vi "Plural Marker.vi"(11 "Size":i32) -> (3 "Plural Mark":string)   [LabVIEW 2021, in "TAF Proj Document Type.lvlib"]
uses:
  <vilib>/Wovalab/AntiDoc/Document Type/Add-ons/LabVIEW TAF Project/TAF Proj Document Type.lvlib
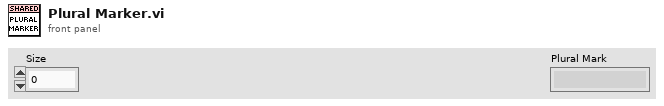
[diagram p1: front panel]
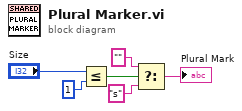
[diagram p0: block diagram]
diagram:
  n1 = Less Or Equal?(x="Size", y=1) -> (x <= y?=w5:bool)
  n2 = Select(t="", s=w5, f="s") -> (s? t:f=→"Plural Mark":string)
